vi "Command_(SubVI).vi"(10 "Команда":u16(ring) items=["0xE0 Запрос количества доступных параметров"=224, "0xE1 Записать один параметр типа float"=225, "0xE2 Записать один параметр типа int"=226, "0xE3 Считать один параметр телеметрии"=227, "0xE4 Записать все параметры типа float"=228, "0xE5 Записать все параметры типа int"=229, "0xE6 Считать все данные телеметрии"=230, "0xE7 Получить описание одного параметра типа float"=231, "0xE8 Получить описание одного параметра типа int"=232, "0xE9 Получить описание одного параметра телеметрии"=233, "0xEA Считать один параметр типа float"=234, "0xEB Считать один параметр типа int"=235, "0xEC Считать все параметры типа float"=236, "0xED Считать все параметры типа int"=237, "0xEE Считать считать фрагмент описания устройства в формате JSON"=238, "0x06 Записать UUID"=6, "0x07 Чтение UUID"=7, "0x45 Считывание параметров Flash памяти"=69, "0x43 Запись страницы Flash памяти"=67, "0x44 Чтения страницы Flash памяти"=68, "0x46 Получить описание Flash-памяти"=70, "0xFA Программный сброс"=250, "0xFB Изменение скорости интерфейса"=251, "0xFF Считывание типа и версии устройства"=255, "0x50 Запрос кол-ва табличных параметров"=80, "0x51 Запрос описания табличного параметра"=81, "0x52 Чтение данных табличного параметра"=82, "0x53 Запись данных табличного параметра"=83, "0x54 Подготовка табличного параметра"=84, "0x55 Запрос прогресса подготовки табличного параметра"=85, "0x56 Освобождение данных подготовленного табличного параметра"=86], 11 "String in":string) -> (3 "String out":string)   [LabVIEW 2017, in "LV_Unicorn.lvlib"]
uses:
  LV_Unicorn.lvlib
  <vilib>/Utility/miscctls.llb/LVStringsAndValuesArrayTypeDef_U16.ctl
panel:
  out "decimal integer string":string
  in  "Strings And Values []":T1=[{"String"="0xE0 Запрос количества доступных параметров", "Value"=224}, {"String"="0xE1 Записать один параметр типа float", "Value"=225}, {"String"="0xE2 Записать один параметр типа int", "Value"=226}, {"String"="0xE3 Считать один параметр телеметрии", "Value"=227}, {"String"="0xE4 Записать все параметры типа float", "Value"=228}, {"String"="0xE5 Записать все параметры типа int", "Value"=229}, {"String"="0xE6 Считать все данные телеметрии", "Value"=230}, {"String"="0xE7 Получить описание одного параметра типа float", "Value"=231}, {"String"="0xE8 Получить описание одного параметра типа int", "Value"=232}, {"String"="0xE9 Получить описание одного параметра телеметрии", "Value"=233}, {"String"="0xEA Считать один параметр типа float", "Value"=234}, {"String"="0xEB Считать один параметр типа int", "Value"=235}, {"String"="0xEC Считать все параметры типа float", "Value"=236}, {"String"="0xED Считать все параметры типа int", "Value"=237}, {"String"="0xEE Считать считать фрагмент описания устройства в формате JSON", "Value"=238}, {"String"="0x06 Записать UUID", "Value"=6}, {"String"="0x07 Чтение UUID", "Value"=7}, {"String"="0x45 Считывание параметров Flash памяти", "Value"=69}, {"String"="0x43 Запись страницы Flash памяти", "Value"=67}, {"String"="0x44 Чтения страницы Flash памяти", "Value"=68}, {"String"="0x46 Получить описание Flash-памяти", "Value"=70}, {"String"="0xFA Программный сброс", "Value"=250}, {"String"="0xFB Изменение скорости интерфейса", "Value"=251}, {"String"="0xFF Считывание типа и версии устройства", "Value"=255}, {"String"="0x50 Запрос кол-ва табличных параметров", "Value"=80}, {"String"="0x51 Запрос описания табличного параметра", "Value"=81}, {"String"="0x52 Чтение данных табличного параметра", "Value"=82}, {"String"="0x53 Запись данных табличного параметра", "Value"=83}, {"String"="0x54 Подготовка табличного параметра", "Value"=84}, {"String"="0x55 Запрос прогресса подготовки табличного параметра", "Value"=85}, {"String"="0x56 Освобождение данных подготовленного табличного параметра", "Value"=86}] {"Value" format="%x"}
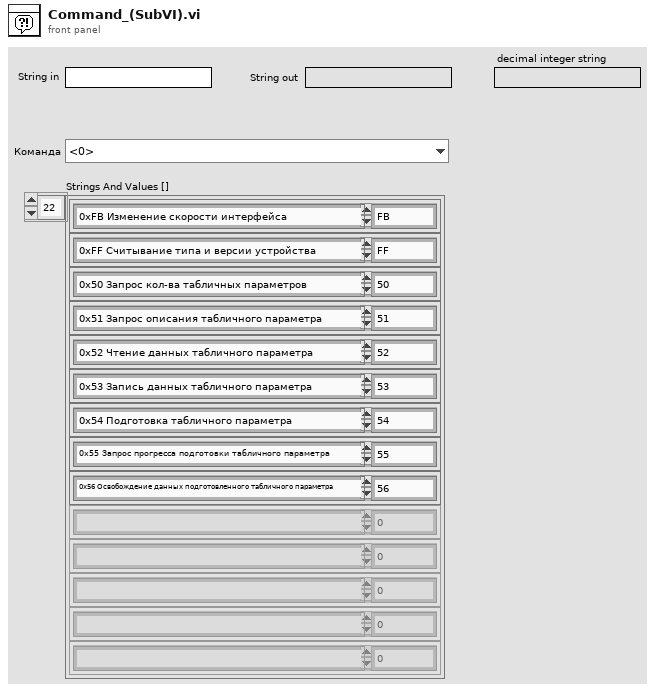
[diagram p1: front panel]
types:
  T1 = typedef "LVStringsAndValuesArrayTypeDef_U16.ctl" = cluster{"String":string, "Value":u16}[]
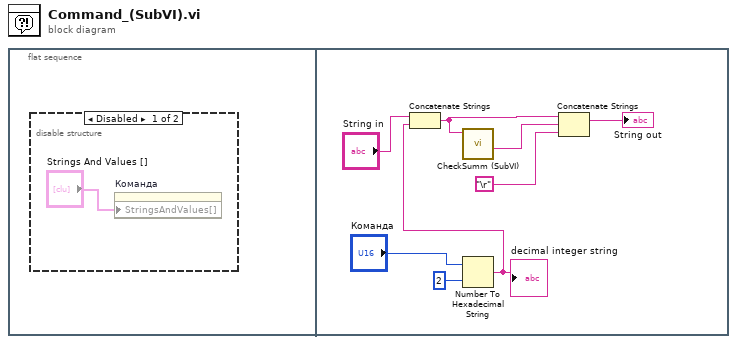
[diagram p0: block diagram]
diagram:
  n1 = flat-sequence {
    frame #0 {
      n2 = disable-structure shown="Disabled" {
        frame Disabled {
          n3 = property on="Команда" class="Ring (strict)"("StringsAndValues[]"="Strings And Values []") -> ()  [unwired: 2 in, 2 out]
        }
        frame Enabled {
        }
      }
    }
    frame #1 {
      n4 = Number To Hexadecimal String(1:i16 2 ("width (-)"), 2:"Команда") -> (0:w2:string)
      "decimal integer string" <- w2
      n5 = Concatenate Strings("String in", w2) -> (w6:string)
      n6 = call "CheckSumm (SubVI).vi"("Input String"=w6) -> ("CheckSumm"=w5:string)  [unwired: 7 in, 3 out]
      n7 = Concatenate Strings(w6, w5, "\r") -> (→"String out":string)
    }
  }
